vi "File to Array.vi"(8 "error in":errorcluster, 11 "file path in":path) -> (0 "error out":errorcluster, 2 "list out":T1[](array[typedef]) {"Creation Date" format="%<%x>T"; "Last Updated" format="%<%x>T"}, 3 "file path out":path)   [LabVIEW 2018]
uses:
  Type Defs/SR Cluster.ctl
  Type Defs/SR Status.ctl
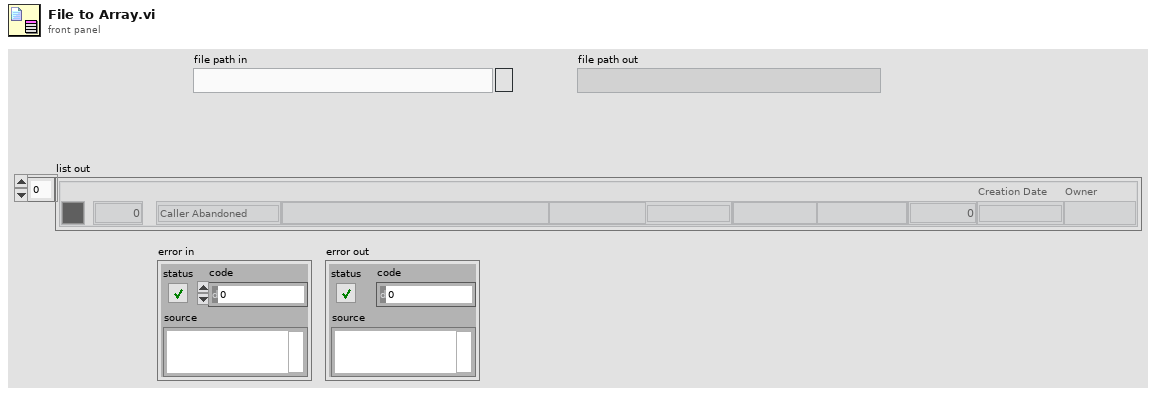
[diagram p1: front panel]
types:
  T1 = typedef "SR Cluster.ctl" = cluster{"Color":u32, "SR Number":i32, "SR Status":T2, "Name":string, "Summary":string, "Last Updated":timestamp, "SR Type":string, "Service Level":string, "Days Open":dbl, "Creation Date":timestamp, "Owner":string}
  T2 = typedef "SR Status.ctl" = enum16{"Caller Abandoned", "Created in Error", "Expired", "Forum Resolved AE", "Forum Resolved Customer", "IN WORK", "IN WORK Collab with AES", "IN WORK Collab with PSE", "IN WORK Collab with SE", "IN WORK Customer Added Note", "IN WORK Escalation", "IN WORK Wait on Customer", "Open", "Potentially Resolved", "Presumed Resolved", "RMA Approved for Return", "RMA Closed", "RMA Closed - DOA", "RMA In Progress", "RMA Open", "RMA Waiting on Customer", "Resolved", "Passed Off"}
  T3 = enum16{"open", "replace", "create", "open or create", "replace or create", "replace or create with confirmation"}
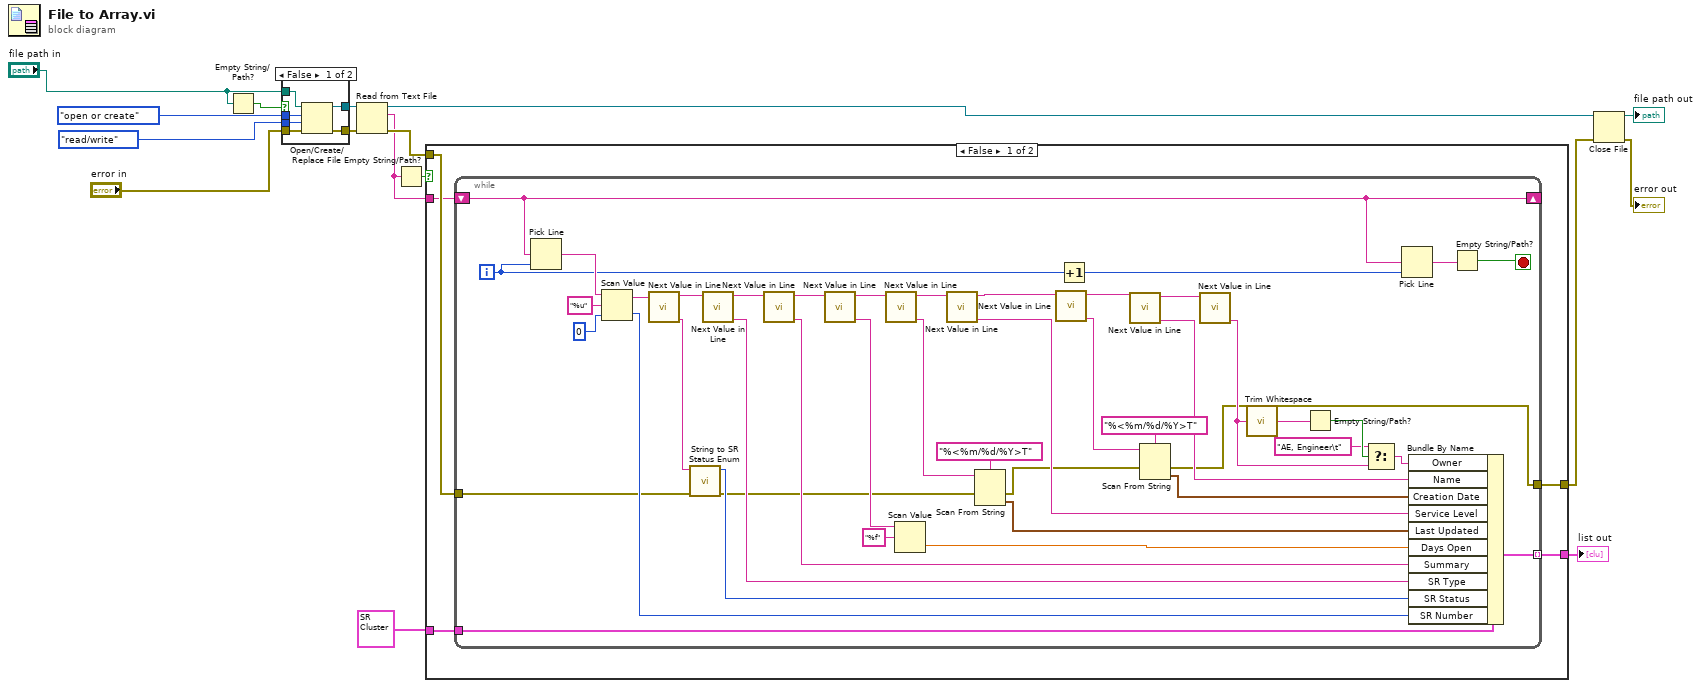
[diagram p0: block diagram]
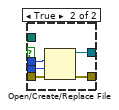
[diagram p2: hidden frame]
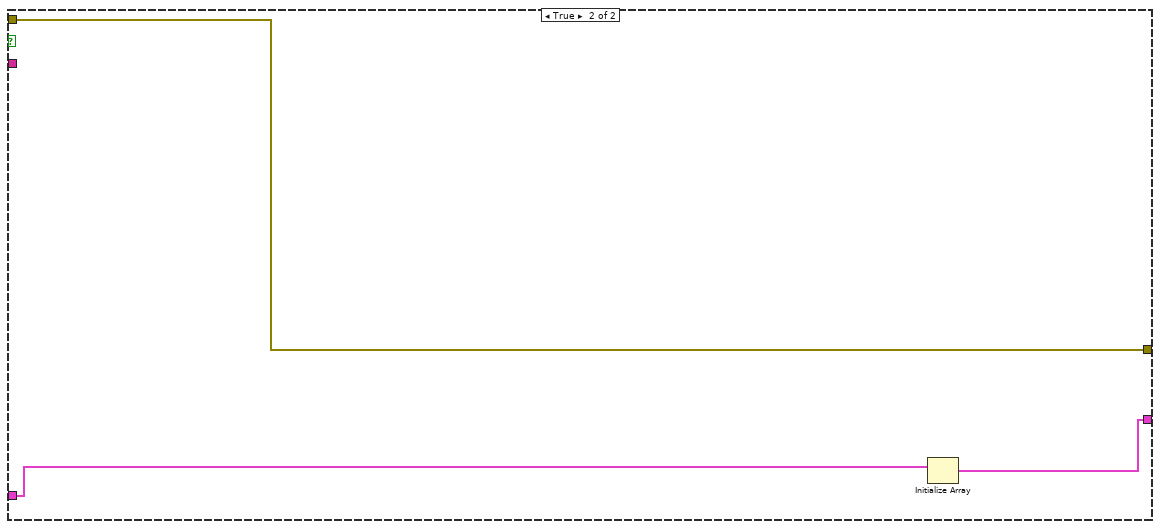
[diagram p3: hidden frame]
diagram:
  n1 = Empty String/Path?(string/path="file path in") -> (empty?=w2:bool)
  n2 = case shown="False" w2 {
    tunnel: enum16{"read/write", "read-only", "write-only"}."read/write" ("access (0:read/write)") -> [w22 w26]
    tunnel: T3."open or create" ("operation (0:open)") -> [w21 w27]
    tunnel: "error in" -> [w20 w25]
    tunnel: [w19 w23] -> w13
    tunnel: [w18 w24] -> w12
    tunnel: "file path in" -> [w17 _]
    frame False {
      n3 = Open/Create/Replace File(file path (use dialog)=w17, error in=w20, operation (0:open)=w21, access (0:read/write)=w22) -> (refnum out=w19:refnum<file>, error out=w18:errorcluster)  [unwired: 2 in, 1 out]
    }
    frame True {
      n4 = Open/Create/Replace File(error in=w25, operation (0:open)=w27, access (0:read/write)=w26) -> (refnum out=w23:refnum<file>, error out=w24:errorcluster)  [unwired: 3 in, 1 out]
    }
  }
  n5 = Read from Text File(file (use dialog)=w13, error in=w12) -> (refnum out=w7:refnum<file>, text=w9:string, error out=w10:errorcluster)  [unwired: 2 in, 1 out]
  n6 = Empty String/Path?(string/path=w9) -> (empty?=w11:bool)
  n7 = case shown="False" w11 {
    tunnel: w10 -> [w31 w77]
    tunnel: w9 -> [w30 _]
    tunnel: T1 {"Color"=0, "SR Number"=0, "SR Status"=enum."Caller Abandoned", "Name"="", "Summary"="", "Last Updated"=timestamp(0 s since 1904-01-01), "SR Type"="", "Service Level"="", "Days Open"=0.0, "Creation Date"=timestamp(0 s since 1904-01-01), "Owner"=""} ("SR Cluster") -> [w32 w79]
    tunnel: [w29 w77] -> w6
    tunnel: [w28 w78] -> w5
    frame False {
      n8 = while {
        tunnel: w32 -> [w67]
        tunnel: w31 -> [w48]
        shift-right: [w55] -> _
        shift-left: w30 -> [w55]
        tunnel: [w56] -> w28 mode=indexing
        tunnel: [w33] -> w29
        i -> [w52]
        stop <- w53 stop-if-true
        n9 = Pick Line(multi-line string=w55, line index=w52) -> (output string=w76:string)  [unwired: 1 in]
        n10 = Scan Value(string=w76, format string="%u", default (0 dbl)=0) -> (output string=w73:string, value=w66:i32)
        n11 = call "Next Value in Line.vi"("string in"=w73) -> ("value"=w50:string, "rest of string"=w72:string)  [unwired: 9 in]
        n12 = call "String to SR Status Enum.vi"("error in"=w48, "string in"=w50) -> ("error out"=w47:errorcluster, "SR Status"=w49:T2)  [unwired: 8 in]
        n13 = call "Next Value in Line.vi"("string in"=w72) -> ("value"=w65:string, "rest of string"=w71:string)  [unwired: 9 in]
        n14 = call "Next Value in Line.vi"("string in"=w71) -> ("value"=w64:string, "rest of string"=w70:string)  [unwired: 9 in]
        n15 = call "Next Value in Line.vi"("string in"=w70) -> ("value"=w62:string, "rest of string"=w69:string)  [unwired: 9 in]
        n16 = call "Next Value in Line.vi"("string in"=w69) -> ("value"=w60:string, "rest of string"=w68:string)  [unwired: 9 in]
        n17 = Scan Value(string=w62, format string="%f") -> (value=w63:dbl)  [unwired: 1 in, 1 out]
        n18 = call "Next Value in Line.vi"("string in"=w68) -> ("value"=w57:string, "rest of string"=w46:string)  [unwired: 9 in]
        n19 = Scan From String(format string="%<%m/%d/%Y>T", input string=w60, error in=w47) -> (error out=w42:errorcluster, output 1=w58:timestamp)  [unwired: 2 in, 2 out]
        n20 = call "Next Value in Line.vi"("string in"=w46) -> ("value"=w45:string, "rest of string"=w41:string)  [unwired: 9 in]
        n21 = Increment(x=w52) -> (x+1=w51:i32)
        n22 = call "Next Value in Line.vi"("string in"=w41) -> ("value"=w40:string, "rest of string"=w39:string)  [unwired: 9 in]
        n23 = Scan From String(format string="%<%m/%d/%Y>T", input string=w45, error in=w42) -> (error out=w33:errorcluster, output 1=w43:timestamp)  [unwired: 2 in, 2 out]
        n24 = call "Next Value in Line.vi"("string in"=w39) -> ("value"=w34:string)  [unwired: 9 in, 1 out]
        n25 = call <vilib>:"Trim Whitespace.vi"("string"=w34) -> ("trimmed string"=w38:string)  [unwired: 1 in]
        n26 = Empty String/Path?(string/path=w38) -> (empty?=w37:bool)
        n27 = Select(t="AE, Engineer\t", s=w37, f=w34) -> (s? t:f=w35:string)
        n28 = Pick Line(multi-line string=w55, line index=w51) -> (output string=w54:string)  [unwired: 1 in]
        n29 = Bundle By Name(cluster=w67, "Owner"=w35, "Name"=w40, "Creation Date"=w43, "Service Level"=w57, "Last Updated"=w58, "Days Open"=w63, "Summary"=w64, "SR Type"=w65, "SR Status"=w49, "SR Number"=w66) -> (w56:T1)
        n30 = Empty String/Path?(string/path=w54) -> (empty?=w53:bool)
      }
    }
    frame True {
      n31 = Initialize Array(w79) -> (w78:T1[])  [unwired: 1 in]
    }
  }
  "list out" <- w5
  n32 = Close File(refnum=w7, error in=w6) -> (path=→"file path out":path, error out=→"error out":errorcluster)
